vi "sv_Check Freq Range.vi"(8 "error in (no error)":errorcluster, 9 "range in":cluster{"start":dbl, "stop":dbl}={"start"=-1.0, "stop"=-1.0} {"stop" format="%.2f"; "start" format="%.2f"}, 10 "octave info in":T1={"standard"=enum."ANSI S1.11", "bandwidth"=enum."1 octave", "low band"=0, "high band"=0, "weighting filter"=0, "dB reference"=0.0, "dB On"=FALSE, "unit label"="", "channel name"="", "description"="", "engineering units"=1, "custom label"="", "spectrum type"=enum."magnitude", "spectral density"=FALSE, "filters settled"=FALSE} {"engineering units" items=["custom..."=0, "V"=1, "A"=21, "C"=30, "pC"=31, "s"=32, "-"=29, "Pa"=2, "N"=20, "g"=3, "m/s^2"=4, "m/s"=5, "m"=6, "mm/s"=12, "mm"=13, "micron/s"=14, "micron"=15, "in/s^2"=7, "in/s"=8, "in"=9, "mil/s"=10, "mil"=11, "rad/s^2"=16, "rad/s"=17, "rad"=18, "deg/s^2"=26, "deg/s"=27, "deg"=28, "RPM"=22, "cycle/s^2"=23, "Hz"=24, "cycle"=25, "strain"=19]; "dB reference" format="%.2e"; "weighting filter" items=["Linear", "A-weighting", "B-weighting", "C-weighting", "ITU-R 468-4", "Dolby", "CCITT", "C-message", "Wb", "Wc", "Wd", "We", "Wf", "Wh", "Wj", "Wk", "Wm", "AES17 20 kHz lowpass", "AES17 40 kHz lowpass", "AES17 20 kHz highpass", "AES17 40 kHz highpass"]}, 11 "nominal frequencies [Hz]":dbl[](array[numeric])) -> (0 "error out":errorcluster, 1 "range out":cluster{"start":dbl, "stop":dbl}={"start"=-1.0, "stop"=-1.0} {"stop" format="%.2f"; "start" format="%.2f"}, 2 "octave info out":T1={"standard"=enum."ANSI S1.11", "bandwidth"=enum."1 octave", "low band"=0, "high band"=0, "weighting filter"=0, "dB reference"=0.0, "dB On"=FALSE, "unit label"="", "channel name"="", "description"="", "engineering units"=1, "custom label"="", "spectrum type"=enum."magnitude", "spectral density"=FALSE, "filters settled"=FALSE} {"engineering units" items=["custom..."=0, "V"=1, "A"=21, "C"=30, "pC"=31, "s"=32, "-"=29, "Pa"=2, "N"=20, "g"=3, "m/s^2"=4, "m/s"=5, "m"=6, "mm/s"=12, "mm"=13, "micron/s"=14, "micron"=15, "in/s^2"=7, "in/s"=8, "in"=9, "mil/s"=10, "mil"=11, "rad/s^2"=16, "rad/s"=17, "rad"=18, "deg/s^2"=26, "deg/s"=27, "deg"=28, "RPM"=22, "cycle/s^2"=23, "Hz"=24, "cycle"=25, "strain"=19]; "dB reference" format="%.2e"; "weighting filter" items=["Linear", "A-weighting", "B-weighting", "C-weighting", "ITU-R 468-4", "Dolby", "CCITT", "C-message", "Wb", "Wc", "Wd", "We", "Wf", "Wh", "Wj", "Wk", "Wm", "AES17 20 kHz lowpass", "AES17 40 kHz lowpass", "AES17 20 kHz highpass", "AES17 40 kHz highpass"]}, 3 "in range?":bool)   [LabVIEW 2017, in "SoundVib_Octave.lvlib"]
doc: "This VI checks if the <B>range in</B> input frequencies are within the low bandedge of the lowest nominal frequency and the high bandedge frenquency of the the highest nominal frequency. It returns errors if the input <B>range in</B> is out of range. It returns a warning if the input <B>range in</B> is coerced. <B>range out</B> corresponds to the range of the nominal frequencies covered by <B>range in</B>. <B>octave info out</B> contains the low and high bands that correspond to <B>range in</B>."
uses:
  <vilib>/addons/Sound and Vibration/svt_Octave/SoundVib_Octave.lvlib
  <vilib>/addons/_NISVFA/_Shared subVIs/Controls/svc_Octave Info.ctl
  <vilib>/addons/_NISVFA/_Shared subVIs/Controls/svc_Octave Standard.ctl
  <vilib>/addons/_NISVFA/_Shared subVIs/Controls/svc_Weighting Filter Text Ring.ctl
  <vilib>/addons/_NISVFA/_Shared subVIs/Controls/svc_Engineering Units Text Ring.ctl
panel:
  out "zero span?":bool
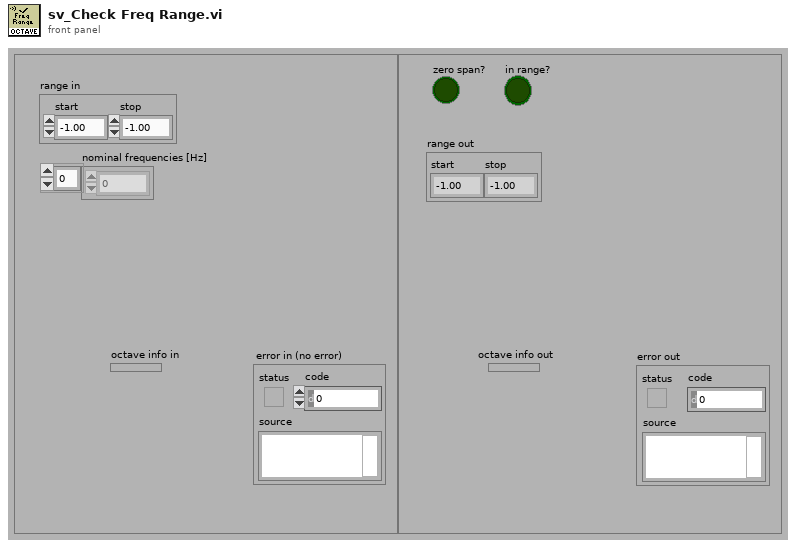
[diagram p1: front panel]
types:
  T1 = typedef "svc_Octave Info.ctl" = cluster{"standard":T2, "bandwidth":enum16{"1 octave", "1/3 octave", "1/6 octave", "1/12 octave", "1/24 octave"}, "low band":i32, "high band":i32, "weighting filter":T3, "dB reference":dbl, "dB On":bool, "unit label":string, "channel name":string, "description":string, "engineering units":T4, "custom label":string, "spectrum type":enum16{"power", "magnitude"}, "spectral density":bool, "filters settled":bool}
  T2 = typedef "svc_Octave Standard.ctl" = enum16{"ANSI S1.11", "IEC 61260"}
  T3 = typedef "svc_Weighting Filter Text Ring.ctl" = u16
  T4 = typedef "svc_Engineering Units Text Ring.ctl" = u16
  T5 = cluster{"f low":dbl, "f high":dbl, "midband":dbl}[]
  T6 = cluster{"f low":dbl, "f high":dbl, "midband":dbl}
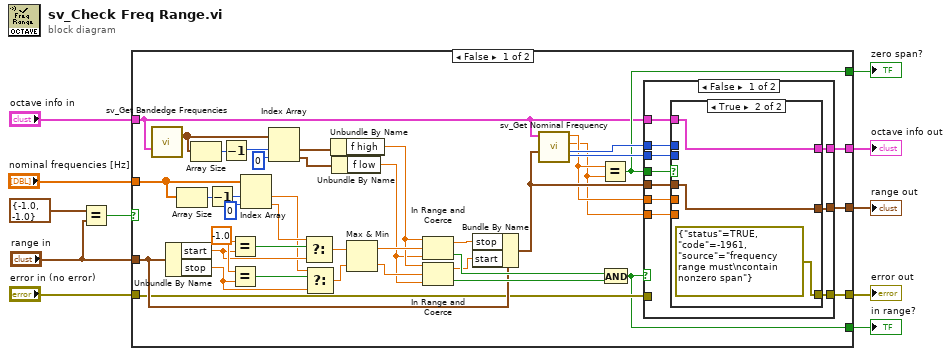
[diagram p0: block diagram]
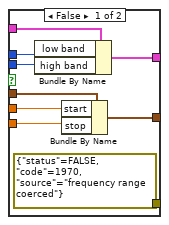
[diagram p2: hidden frame]
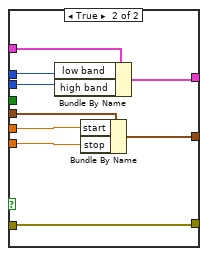
[diagram p3: hidden frame]
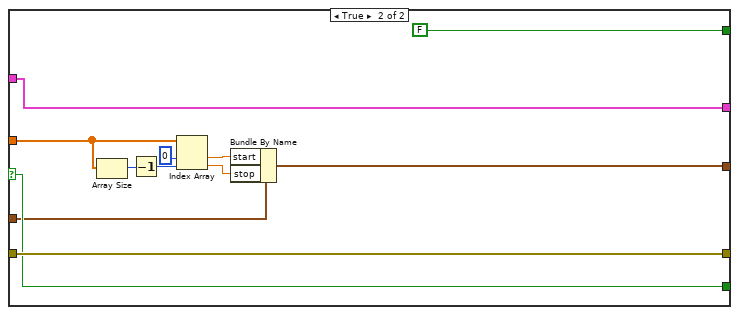
[diagram p4: hidden frame]
diagram:
  n1 = Equal?(x=cluster{"start":dbl, "stop":dbl} {"start"=-1.0, "stop"=-1.0} ("range"), y="range in") -> (x = y?=w10:bool)
  n2 = case shown="False" w10 {
    selector: w10 -> [_ w93]
    tunnel: "nominal frequencies [Hz]" -> [w51 w91]
    tunnel: [w34 w94] -> w2
    tunnel: "range in" -> [w36 w86]
    tunnel: [w22 w93] -> w4
    tunnel: "error in (no error)" -> [w35 w94]
    tunnel: [w32 w85] -> w6
    tunnel: [w21 FALSE] -> w5
    tunnel: "octave info in" -> [w20 w83]
    tunnel: [w29 w83] -> w1
    frame False {
      w49 = -1.0 ("x")
      n3 = call <vilib>:"sv_Get Bandedge Frequencies.vi"("octave info"=w20) -> ("bandedge frequencies [Hz]"=w16:T5)  [unwired: 13 in, 1 out]
      n4 = Unbundle By Name(w36) -> ("start"=w44:dbl, "stop"=w45:dbl)
      n5 = Array Size(array=w51) -> (size(s)=w50:i32)
      n6 = Array Size(array=w16) -> (size(s)=w19:i32)
      n7 = Decrement(x=w50) -> (x-1=w42:i32)
      n8 = Decrement(x=w19) -> (x-1=w18:i32)
      n9 = Equal?(x=w49, y=w44) -> (x = y?=w47:bool)
      n10 = Equal?(x=w49, y=w45) -> (x = y?=w46:bool)
      n11 = Index Array(array=w51, index #1=w42, index #2=0 ("index")) -> (element #1=w39:dbl, element #2=w40:dbl)
      n12 = Index Array(array=w16, index #1=w18, index #2=0 ("index")) -> (element #1=w15:T6, element #2=w14:T6)
      n13 = Select(t=w40, s=w47, f=w44) -> (s? t:f=w48:dbl)
      n14 = Select(t=w39, s=w46, f=w45) -> (s? t:f=w43:dbl)
      n15 = Unbundle By Name(w15) -> ("f high"=w13:dbl)
      n16 = Unbundle By Name(w14) -> ("f low"=w12:dbl)
      n17 = Max & Min(x=w48, y=w43) -> (max(x,y)=w28:dbl, min(x,y)=w27:dbl)
      n18 = In Range and Coerce(upper limit=w13, x=w28, lower limit=w12) -> (coerced(x)=w26:dbl, In Range?=w38:bool)
      n19 = In Range and Coerce(upper limit=w13, x=w27, lower limit=w12) -> (coerced(x)=w24:dbl, In Range?=w37:bool)
      n20 = Bundle By Name(cluster=w36, "stop"=w26, "start"=w24) -> (w33:cluster{"start":dbl, "stop":dbl})
      n21 = call <vilib>:"sv_Get Nominal Frequency.vi"("frequency range [Hz]"=w33, "octave info"=w20) -> ("high band"=w30:i32, "low band"=w31:i32, "high nominal frequency [Hz]"=w23:dbl, "low nominal frequency [Hz]"=w25:dbl)  [unwired: 5 in]
      n22 = Equal?(x=w25, y=w23) -> (x = y?=w21:bool)
      n23 = And(x=w38, y=w37) -> (x .and. y?=w22:bool)
      n24 = case shown="False" w22 {
        tunnel: w35 -> [_ w82]
        tunnel: [w61 w82] -> w34
        tunnel: w33 -> [w60 w81]
        tunnel: w25 -> [w59 w80]
        tunnel: w23 -> [w58 w79]
        tunnel: [w57 w78] -> w32
        tunnel: w20 -> [w56 w74]
        tunnel: w31 -> [w55 w77]
        tunnel: w30 -> [w54 w76]
        tunnel: [w53 w75] -> w29
        tunnel: w21 -> [w52 _]
        frame False {
          n25 = case shown="True" w52 {
            tunnel: [errorcluster {"status"=FALSE, "code"=1970, "source"="frequency range coerced"} ("error in (no error)") errorcluster {"status"=TRUE, "code"=-1961, "source"="frequency range must\ncontain nonzero span"} ("error in (no error)")] -> w61
            tunnel: w60 -> [w69 w72]
            tunnel: w59 -> [w68 _]
            tunnel: w58 -> [w67 _]
            tunnel: [w66 w72] -> w57
            tunnel: w56 -> [w65 w71]
            tunnel: w55 -> [w64 _]
            tunnel: w54 -> [w63 _]
            tunnel: [w62 w71] -> w53
            frame False {
              n26 = Bundle By Name(cluster=w65, "low band"=w64, "high band"=w63) -> (w62:T1)
              n27 = Bundle By Name(cluster=w69, "start"=w68, "stop"=w67) -> (w66:cluster{"start":dbl, "stop":dbl})
            }
            frame True {
            }
          }
        }
        frame True {
          # "in range"
          n28 = Bundle By Name(cluster=w74, "low band"=w77, "high band"=w76) -> (w75:T1)
          n29 = Bundle By Name(cluster=w81, "start"=w80, "stop"=w79) -> (w78:cluster{"start":dbl, "stop":dbl})
        }
      }
    }
    frame True {
      n30 = Array Size(array=w91) -> (size(s)=w84:i32)
      n31 = Decrement(x=w84) -> (x-1=w90:i32)
      n32 = Index Array(array=w91, index #1=0 ("index"), index #2=w90) -> (element #1=w88:dbl, element #2=w87:dbl)
      n33 = Bundle By Name(cluster=w86, "start"=w88, "stop"=w87) -> (w85:cluster{"start":dbl, "stop":dbl})
    }
  }
  "error out" <- w2
  "in range?" <- w4
  "range out" <- w6
  "zero span?" <- w5
  "octave info out" <- w1
